vi "XY Graph Is Grid Hidden.vi"(8 "Error In":errorcluster, 11 "XY Graph Ref":T1) -> (0 "Error Out (dup)":errorcluster, 1 "Hidden Grid(s)":bool)   [LabVIEW 2019, in "XY Graph Add-Ons.lvlib"]
uses:
  XY Graph Add-Ons.lvlib
  XY Graph Refnum.ctl
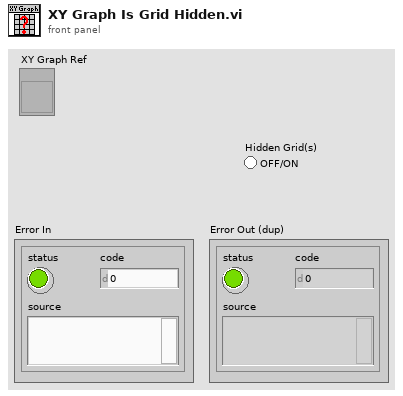
[diagram p1: front panel]
types:
  T1 = typedef "XY Graph Add-Ons.lvlib/XY Graph Refnum.ctl" = refnum<vi>
  T2 = typedef "LVMajorAndMinorColorsTypeDef.ctl" = cluster{"Major Color":u32, "Minor Color":u32}
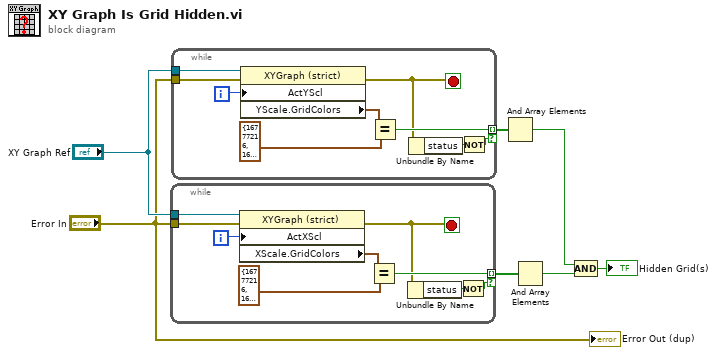
[diagram p0: block diagram]
diagram:
  n1 = while {
    tunnel: "Error In" -> [w15]
    tunnel: [w12] -> w7 mode=indexing if=w8
    tunnel: "XY Graph Ref" -> [w16]
    i -> [w11]
    stop <- w10 stop-if-true
    n2 = property class="XYGraph (strict)"(reference=w16, error in=w15, "ActXScl"=w11) -> (error out=w10:errorcluster, "XScale.GridColors"=w14:T2)  [unwired: 1 out]
    n3 = Equal?(x=w14, y=cluster{"Major Color":u32, "Minor Color":u32} {"Major Color"=16777216, "Minor Color"=16777216} ("X Scale.Grid Colors")) -> (x = y?=w12:bool)
    n4 = Unbundle By Name(w10) -> ("status"=w9:bool)
    n5 = Not(x=w9) -> (.not. x?=w8:bool)
  }
  n6 = while {
    tunnel: "Error In" -> [w24]
    tunnel: [w21] -> w2 mode=indexing if=w17
    tunnel: "XY Graph Ref" -> [w25]
    i -> [w20]
    stop <- w19 stop-if-true
    n7 = property class="XYGraph (strict)"(reference=w25, error in=w24, "ActYScl"=w20) -> (error out=w19:errorcluster, "YScale.GridColors"=w23:T2)  [unwired: 1 out]
    n8 = Equal?(x=w23, y=cluster{"Major Color":u32, "Minor Color":u32} {"Major Color"=16777216, "Minor Color"=16777216} ("X Scale.Grid Colors")) -> (x = y?=w21:bool)
    n9 = Unbundle By Name(w19) -> ("status"=w18:bool)
    n10 = Not(x=w18) -> (.not. x?=w17:bool)
  }
  n11 = And Array Elements(Boolean array=w2) -> (logical AND=w5:bool)
  n12 = And Array Elements(Boolean array=w7) -> (logical AND=w4:bool)
  n13 = Compound Arithmetic op=AND(w5, w4) -> (→"Hidden Grid(s)":bool)
  "Error Out (dup)" <- "Error In"
